vi "Frame Get Sound.vi"(8 "error in (no error)":errorcluster, 11 "IDE simple in":refnum<class "Main Panel.lvclass">) -> (0 "error out":errorcluster, 2 "Sound String":string, 3 "IDE simple out":refnum<class "Main Panel.lvclass">)   [LabVIEW 2018, in "Main Panel.lvlib" / "Main Panel.lvclass"]
uses:
  Main Panel.lvclass
  Main Panel.lvclass/Main Panel.ctl
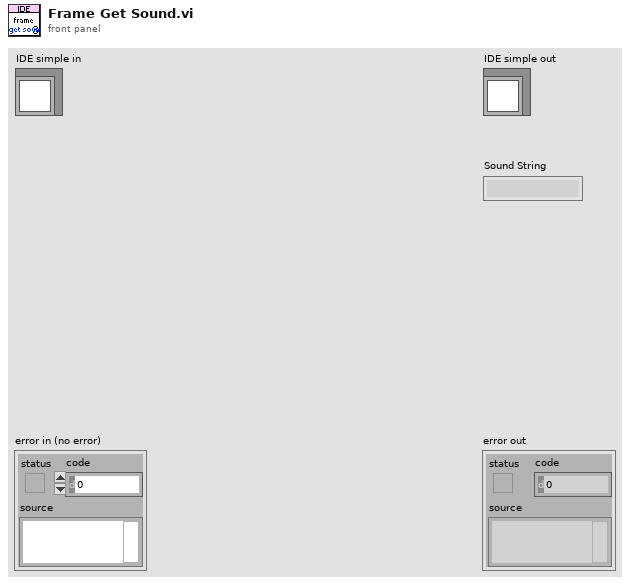
[diagram p1: front panel]
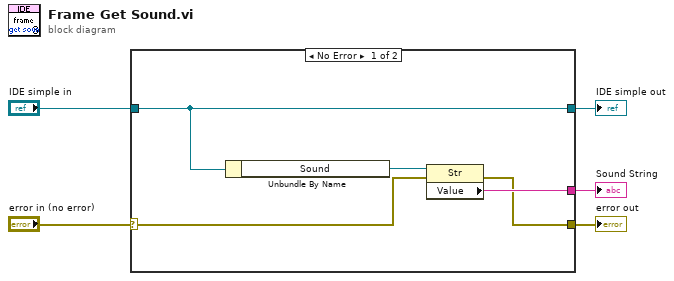
[diagram p0: block diagram]
diagram:
  n1 = case shown="No Error" "error in (no error)" {
    selector: "error in (no error)" -> [w6 w12]
    tunnel: [w7 w12] -> w4
    tunnel: [w10 w11] -> w2
    tunnel: "IDE simple in" -> [w10 w11]
    tunnel: [w8 _] -> w1
    frame No Error {
      n2 = Unbundle By Name(w10) -> ("Sound"=w9:refnum<vi>)
      n3 = property class="Str"(reference=w9, error in=w6) -> (error out=w7:errorcluster, "Value"=w8:string)  [unwired: 1 out]
    }
    frame Error {
    }
  }
  "error out" <- w4
  "IDE simple out" <- w2
  "Sound String" <- w1
